vi "INA219 Init & Config.vi"(7 "I2C Channel":u8, 8 "error in (no error)":errorcluster, 9 "INA219 Config Options":T1={"Reset bit"=0, "Bus Voltage Range"=1, "PGA/Shunt Voltage Gain"=3, "Bus Voltage ADC Settings"=8, "Shunt Voltage ADC Settings"=3, "Mode"=7, "Calibration Value"=4096} {"Calibration Value" format="%.0x"; "Mode" items=["Power Down", "Shunt Voltage, Triggered", "Bus Voltage, Triggered", "Shunt & Bus, Triggered", "ADC Off (Disabled)", "Shunt Voltage, Continuous", "Bus Voltage, Continuous", "Shunt & Bus Voltage, Continuous"]; "Shunt Voltage ADC Settings" items=["9-bit, 84us conversion time"=0, "10-bit, 148us conversion time"=1, "11-bit, 276us conversion time"=2, "12-bit, 532us conversion time"=3, "1x12-bit, 532us conversion time"=8, "2x12-bit averaged, 1.06ms conversion time"=9, "4x12-bit averaged, 2.13ms conversion time"=10, "8x12-bit averaged, 4.26ms conversion time"=11, "16x12-bit averaged, 8.51ms conversion time"=12, "32x12-bit averaged, 17.02ms conversion time"=13, "64x12-bit averaged, 34.05ms conversion time"=14, "128x12-bit averaged, 68.10ms conversion time"=15]; "Bus Voltage ADC Settings" items=["9-bit, 84us conversion time"=0, "10-bit, 148us conversion time"=1, "11-bit, 276us conversion time"=2, "12-bit, 532us conversion time"=3, "1x12-bit, 532us conversion time"=8, "2x12-bit averaged, 1.06ms conversion time"=9, "4x12-bit averaged, 2.13ms conversion time"=10, "8x12-bit averaged, 4.26ms conversion time"=11, "16x12-bit averaged, 8.51ms conversion time"=12, "32x12-bit averaged, 17.02ms conversion time"=13, "64x12-bit averaged, 34.05ms conversion time"=14, "128x12-bit averaged, 68.10ms conversion time"=15]; "PGA/Shunt Voltage Gain" items=["Gain 1, +/-40mV", "Gain 2, +/-80mV", "Gain 3, +/-160mV", "Gain 4, +/-320mV"]; "Bus Voltage Range" items=["0-16V Range", "0-32V Range"]; "Reset bit" items=["Do Not Reset", "Reset"]}, 10 "I2C Slave Address":u8=64 format="%.0x", 11 "LINX Resource in":T2) -> (0 "error out":errorcluster, 1 "INA219 Config Options":T1={"Reset bit"=0, "Bus Voltage Range"=0, "PGA/Shunt Voltage Gain"=0, "Bus Voltage ADC Settings"=0, "Shunt Voltage ADC Settings"=0, "Mode"=0, "Calibration Value"=4096} {"Calibration Value" format="%.0x"; "Mode" items=["Power Down", "Shunt Voltage, Triggered", "Bus Voltage, Triggered", "Shunt & Bus, Triggered", "ADC Off (Disabled)", "Shunt Voltage, Continuous", "Bus Voltage, Continuous", "Shunt & Bus Voltage, Continuous"]; "Shunt Voltage ADC Settings" items=["9-bit, 84us conversion time"=0, "10-bit, 148us conversion time"=1, "11-bit, 276us conversion time"=2, "12-bit, 532us conversion time"=3, "1x12-bit, 532us conversion time"=8, "2x12-bit averaged, 1.06ms conversion time"=9, "4x12-bit averaged, 2.13ms conversion time"=10, "8x12-bit averaged, 4.26ms conversion time"=11, "16x12-bit averaged, 8.51ms conversion time"=12, "32x12-bit averaged, 17.02ms conversion time"=13, "64x12-bit averaged, 34.05ms conversion time"=14, "128x12-bit averaged, 68.10ms conversion time"=15]; "Bus Voltage ADC Settings" items=["9-bit, 84us conversion time"=0, "10-bit, 148us conversion time"=1, "11-bit, 276us conversion time"=2, "12-bit, 532us conversion time"=3, "1x12-bit, 532us conversion time"=8, "2x12-bit averaged, 1.06ms conversion time"=9, "4x12-bit averaged, 2.13ms conversion time"=10, "8x12-bit averaged, 4.26ms conversion time"=11, "16x12-bit averaged, 8.51ms conversion time"=12, "32x12-bit averaged, 17.02ms conversion time"=13, "64x12-bit averaged, 34.05ms conversion time"=14, "128x12-bit averaged, 68.10ms conversion time"=15]; "PGA/Shunt Voltage Gain" items=["Gain 1, +/-40mV", "Gain 2, +/-80mV", "Gain 3, +/-160mV", "Gain 4, +/-320mV"]; "Bus Voltage Range" items=["0-16V Range", "0-32V Range"]; "Reset bit" items=["Do Not Reset", "Reset"]}, 3 "LINX Resource out":T2)   [LabVIEW 2014]
uses:
  <vilib>/MakerHub/LINX/Private/Type Defs/LINX Ref.ctl
  <vilib>/MakerHub/LINX/Private/Type Defs/Platform.ctl
  <vilib>/MakerHub/LINX/Private/Type Defs/Interface.ctl
  <vilib>/MakerHub/LINX/Private/Device/Type Defs/LINX Device Config.ctl
  <vilib>/MakerHub/LINX/Private/Device/Type Defs/TCP Config.ctl
  <vilib>/MakerHub/LINX/Private/Device/Type Defs/Channels.ctl
  INA219 Config Options.ctl
  <vilib>/MakerHub/LINX/Private/Local IO/LinxI2cWrite.vi
  <vilib>/MakerHub/LINX/Public/Utilities/Check Channel.vi
  <vilib>/MakerHub/LINX/Private/Utilties/Generate Error.vi
  <vilib>/MakerHub/LINX/LMH-LINX.lvlib
  <vilib>/MakerHub/LINX/Private/Device/Device.lvlib
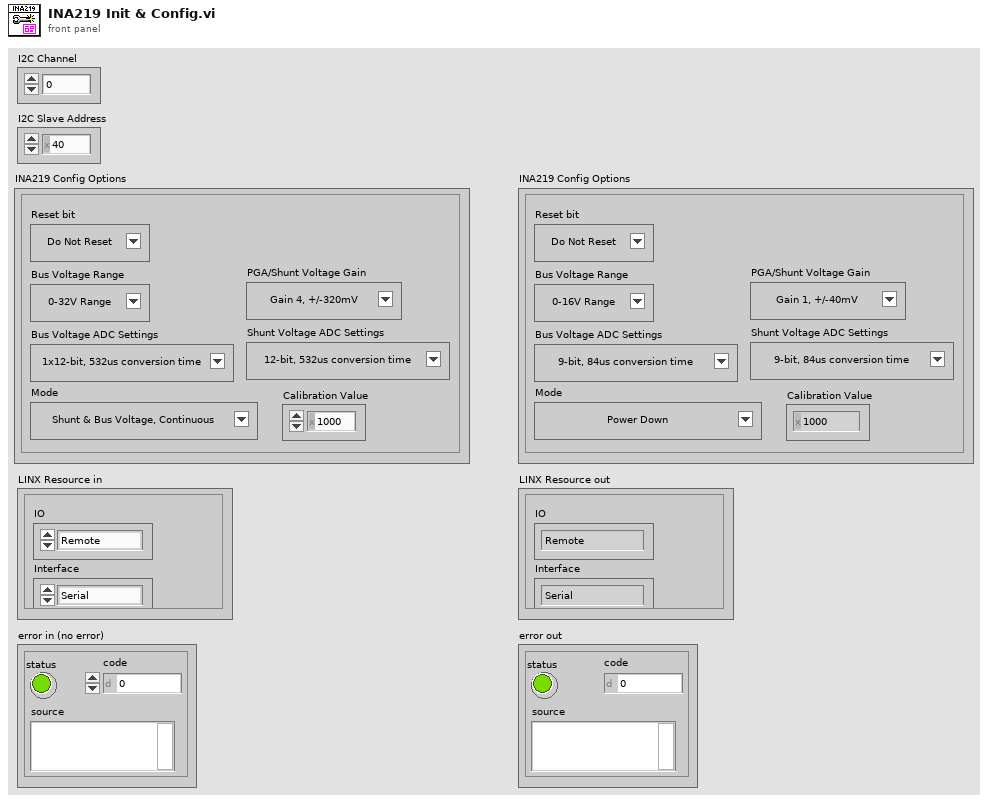
[diagram p1: front panel]
types:
  T1 = typedef "INA219 Config Options.ctl" = cluster{"Reset bit":u8, "Bus Voltage Range":u8, "PGA/Shunt Voltage Gain":u8, "Bus Voltage ADC Settings":u8, "Shunt Voltage ADC Settings":u8, "Mode":u8, "Calibration Value":u16}
  T2 = typedef "LMH-LINX.lvlib/LINX Ref.ctl" = cluster{"IO":T3, "Interface":T4, "LINX Device Config":T5}
  T3 = typedef "LMH-LINX.lvlib/Platform.ctl" = enum16{"Remote", "Local"}
  T4 = typedef "LMH-LINX.lvlib/Interface.ctl" = enum16{"Serial", "TCP"}
  T5 = typedef "LMH-LINX.lvlib/Device.lvlib/LINX Device Config.ctl" = cluster{"Interface":T4, "COM Port":refnum<visa-resource-name>, "TCP Configuration":T6, "Device Family":u8, "Device ID":u8, "Device Name":string, "TCP Ref":refnum<k5>, "Channels":T7}
  T6 = typedef "LMH-LINX.lvlib/Device.lvlib/TCP Config.ctl" = cluster{"IP Address":string, "Port":u16}
  T7 = typedef "LMH-LINX.lvlib/Channels.ctl" = cluster{"DI":u8[], "DO":u8[], "AI":u8[], "AO":u8[], "PWM":u8[], "QE":u8[], "UART":u8[], "I2C 2":u8[], "SPI":u8[], "CAN":u8[], "Servo":u8[], "AI Ref (V)":dbl, "AI Resolution (Bits)":u8, "AO Ref (V)":dbl, "AO Resolution (Bits)":u8}
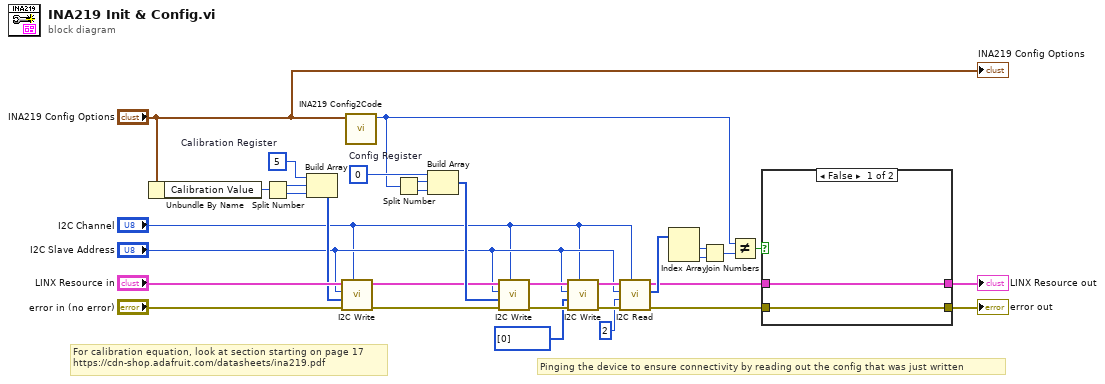
[diagram p0: block diagram]
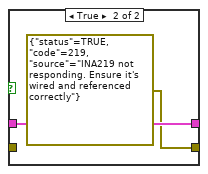
[diagram p2: hidden frame]
diagram:
  w30 = u8 5  # Calibration Register
  w32 = u8 0  # Config Register
  # "Pinging the device to ensure connectivity by reading out the config that was just written"
  # "For calibration equation, look at section starting on page 17\nhttps://cdn-shop.adafruit.com/datasheets/ina219.pdf"
  n1 = Unbundle By Name("INA219 Config Options") -> ("Calibration Value"=w20:u16)
  n2 = Split Number(x=w20) -> (hi(x)=w27:u8, lo(x)=w26:u8)
  n3 = Build Array(w30, w27, w26) -> (w23:u8[])
  n4 = call <vilib>:"I2C Write.vi"("I2C Channel"="I2C Channel", "Error In"="error in (no error)", "Data"=w23, "I2C Slave Address (0)"="I2C Slave Address", "LINX Resource"="LINX Resource in") -> ("Error Out"=w21:errorcluster, "LINX Resource"=w22:T2)  [unwired: 5 in]
  n5 = call "INA219 Config2Code.vi"("INA219 Config Options"="INA219 Config Options") -> ("Config Code"=w7:u16)  [unwired: 10 in]
  n6 = Split Number(x=w7) -> (hi(x)=w28:u8, lo(x)=w29:u8)
  n7 = Build Array(w32, w28, w29) -> (w31:u8[])
  n8 = call <vilib>:"I2C Write.vi"("I2C Channel"="I2C Channel", "Error In"=w21, "Data"=w31, "I2C Slave Address (0)"="I2C Slave Address", "LINX Resource"=w22) -> ("Error Out"=w17:errorcluster, "LINX Resource"=w18:T2)  [unwired: 5 in]
  n9 = call <vilib>:"I2C Write.vi"("I2C Channel"="I2C Channel", "Error In"=w17, "Data"=u8[] [0], "I2C Slave Address (0)"="I2C Slave Address", "LINX Resource"=w18) -> ("Error Out"=w14:errorcluster, "LINX Resource"=w15:T2)  [unwired: 5 in]
  n10 = call <vilib>:"I2C Read.vi"("I2C Channel"="I2C Channel", "Error In"=w14, "Bytes To Read"=u8 2, "I2C Slave Address (0)"="I2C Slave Address", "LINX Resource"=w15) -> ("Error Out"=w4:errorcluster, "Data"=w11:u8[], "LINX Resource"=w6:T2)  [unwired: 4 in]
  n11 = Index Array(array=w11) -> (element #1=w9:u8, element #2=w10:u8)  [unwired: 2 in]
  n12 = Join Numbers(hi=w9, lo=w10) -> ((hi.lo)=w8:u16)
  n13 = Not Equal?(x=w7, y=w8) -> (x != y?=w2:bool)
  n14 = case shown="False" w2 {
    tunnel: w6 -> [w33 w36]
    tunnel: [w33 w36] -> w5
    tunnel: w4 -> [w34 _]
    tunnel: [w34 errorcluster {"status"=TRUE, "code"=219, "source"="INA219 not responding. Ensure it's wired and referenced correctly"} ("error constant")] -> w3
    frame False {
    }
    frame True {
    }
  }
  "error out" <- w3
  "LINX Resource out" <- w5
  "INA219 Config Options" <- "INA219 Config Options"
